vi "Write Temp.vi"(8 "error in (no error)":errorcluster, 10 "Temp":dbl, 11 "Laser State Data in":refnum<class "Laser State Data.lvclass">) -> (0 "error out":errorcluster, 3 "Laser State Data out":refnum<class "Laser State Data.lvclass">)   [LabVIEW 2022 SP3, in "Laser State Data.lvclass"]
uses:
  Laser State Data.lvclass
  Laser State Data.lvclass/Laser State Data.ctl
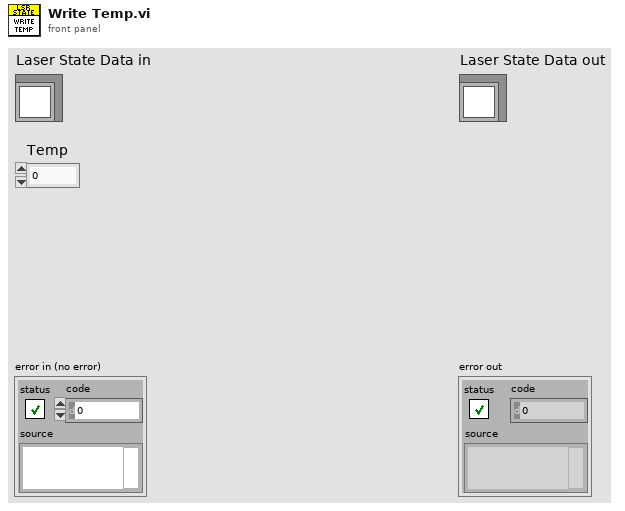
[diagram p1: front panel]
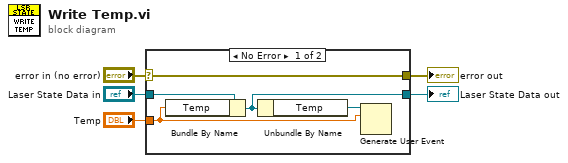
[diagram p0: block diagram]
diagram:
  n1 = case shown="No Error" "error in (no error)" {
    selector: "error in (no error)" -> [w10 w11]
    tunnel: [w10 w11] -> w4
    tunnel: [w7 w12] -> w2
    tunnel: "Laser State Data in" -> [w9 w12]
    tunnel: "Temp" -> [w6 _]
    frame No Error {
      n2 = Bundle By Name(cluster=w9, "Temp"=w6) -> (w7:refnum<class "Laser State Data.lvclass">)
      n3 = Unbundle By Name(w7) -> ("Temp"=w8:refnum<user-event>)
      n4 = Generate User Event(user event=w8, event data cluster=w6) -> ()  [unwired: 2 in, 2 out]
    }
    frame Error {
    }
  }
  "error out" <- w4
  "Laser State Data out" <- w2
